vi "PDash Add Helper Loop.vi"(8 "error in":errorcluster, 10 "Current Selection":T1, 11 "Project":refnum<class "Project.lvclass">) -> (0 "error out":errorcluster, 2 "Current Selection Out":T1, 3 "Project Out":refnum<class "Project.lvclass">)   [LabVIEW 2020, in "Panther Dashboard.lvlib"]
doc: "Panther Dashboard DQMH UI Template"
uses:
  Panther Dashboard.lvlib
  Class/Project/Project.lvclass
  Class/Library/Library.lvclass
  Class/VI/VI.lvclass
  <vilib>/Delacor/Delacor QMH/Libraries/_Scripting Support/Module Type--enum.ctl
  <vilib>/Delacor/Delacor QMH/Libraries/_Scripting Support/dqmh_lib_DQMH Scripting Support.lvlib
  <vilib>/Delacor/Delacor QMH/Libraries/_Scripting Support/Module Info--cluster.ctl
  Controls/Cancel.ctl
  Controls/Continue.ctl
  Controls/Listbox.ctl
panel:
  in  "Current Helper Loops":T2
  out "Selected Module":string caption="Current Module Selection:"
  in  "Helper Loop Name":string
  in  "Continue":T3
  in  "Cancel":T4
  # "Note: To Select the DQMH Default UIs, click the Gear Icon on the Panther Dashboard\nMain UI, and Uncheck the 'Use Panther Dashboard UIs' checkbox."
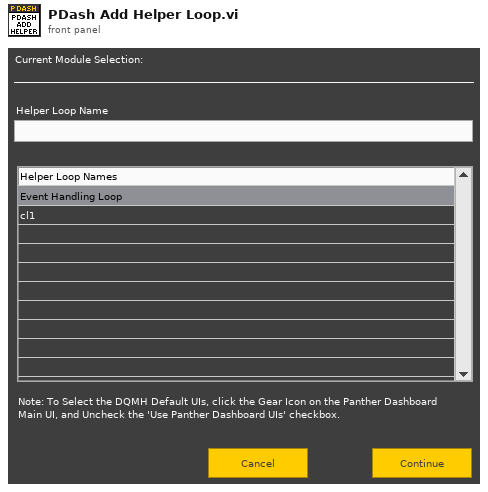
[diagram p1: front panel]
types:
  T1 = cluster{"Library":refnum<class "Library.lvclass">, "VI":refnum<class "VI.lvclass">}
  T2 = typedef "Listbox.ctl" = i32
  T3 = typedef "Continue.ctl" = bool
  T4 = typedef "Cancel.ctl" = bool
  T5 = typedef "dqmh_lib_DQMH Scripting Support.lvlib/Module Info--cluster.ctl" = cluster{"Name":string, "Library":refnum<vi>, "Library Owning App":refnum<vi>, "Library Owning Folder":path, "Module Type":T6, "Public API Requests Folder":refnum<vi>, "Public API Requests Arguments Folder":refnum<vi>, "Broadcasts Folder":refnum<vi>, "Broadcasts Arguments Folder":refnum<vi>, "Obtain Broadcast Events VI":refnum<vi>, "Destroy Broadcast Events VI":refnum<vi>, "Obtain Request Events VI":refnum<vi>, "Destroy Request Events VI":refnum<vi>, "Request Events Cluster CTL":refnum<vi>, "Broadcast Events Cluster CTL":refnum<vi>, "Module Timeout VI":refnum<vi>, "Module Name VI":refnum<vi>, "Status Updated VI":refnum<vi>, "Module Not Running Error Constant VI":refnum<vi>}
  T6 = typedef "dqmh_lib_DQMH Scripting Support.lvlib/Module Type--enum.ctl" = enum16{"Singleton", "Cloneable"}
  T7 = typedef "Panther Dashboard.lvlib/Module type--enum.ctl" = enum16{"Singleton", "Cloneable"}
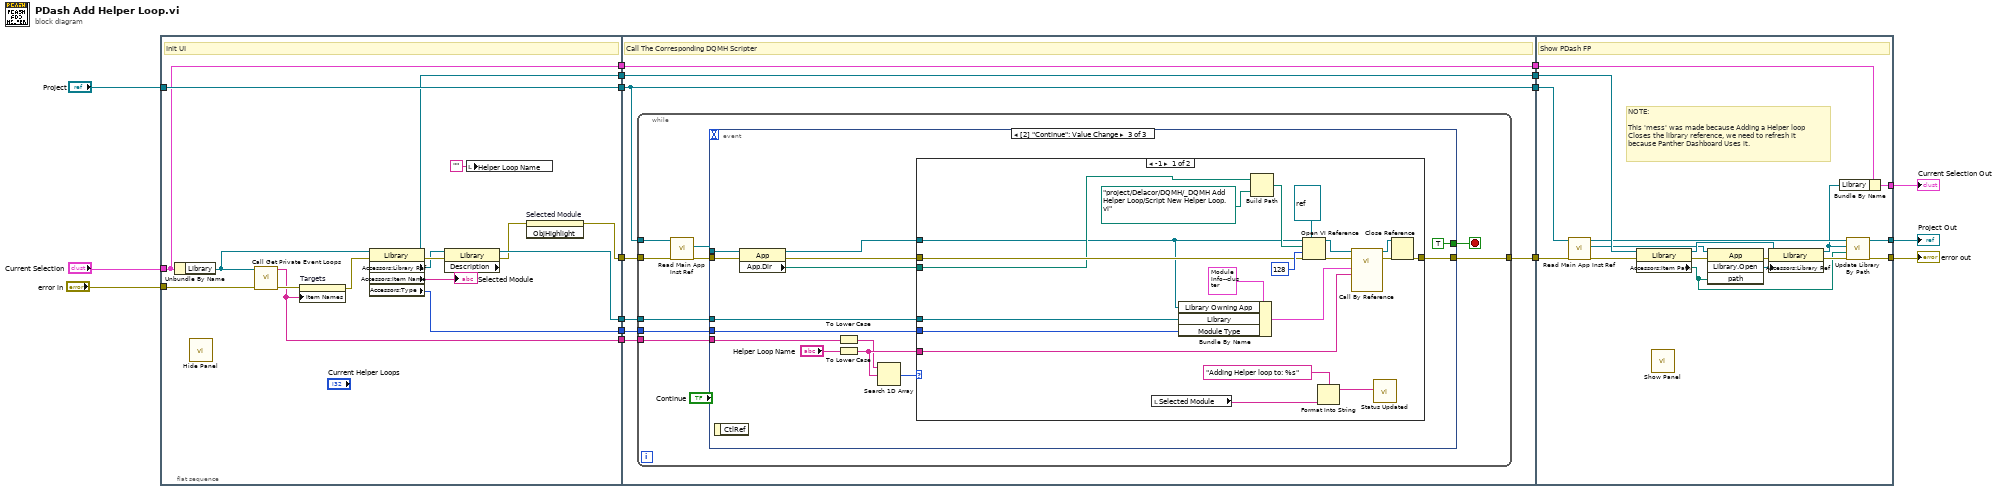
[diagram p0: block diagram]
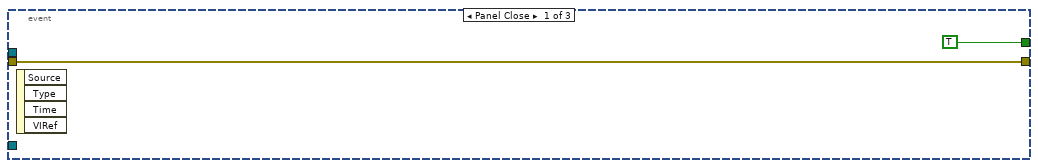
[diagram p2: hidden frame]
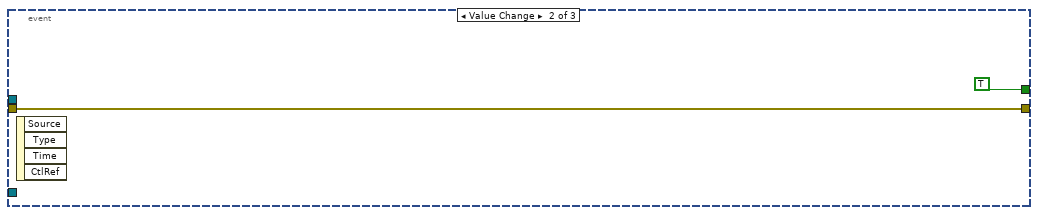
[diagram p3: hidden frame]
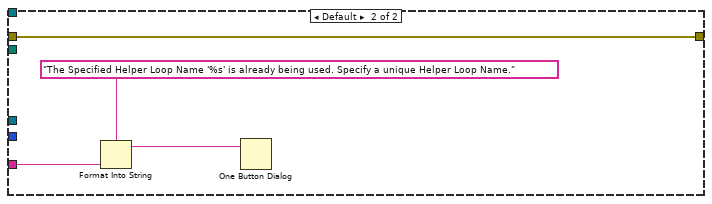
[diagram p4: hidden frame]
diagram:
  n1 = flat-sequence {
    tunnel: "Project" -> [w32]
    tunnel: [w32] -> w13
    tunnel: "error in" -> [w25]
    tunnel: [w26] -> w15
    tunnel: "Current Selection" -> [w20]
    tunnel: [w29] -> w11
    tunnel: [w22] -> w10
    tunnel: [w21] -> w9
    tunnel: [w20] -> w6
    tunnel: [w18] -> w4
    tunnel: [w41] -> w17
    tunnel: w13 -> [w34]
    tunnel: w15 -> [w40]
    tunnel: w11 -> [w39]
    tunnel: w10 -> [w38]
    tunnel: w9 -> [w37]
    tunnel: [w36] -> w7
    tunnel: w6 -> [w36]
    tunnel: w4 -> [w35]
    tunnel: [w35] -> w3
    tunnel: [w34] -> w1
    tunnel: [w100] -> w8
    tunnel: w17 -> [w97]
    tunnel: [w108] -> w5
    tunnel: w7 -> [w109]
    tunnel: w3 -> [w104]
    tunnel: [w102] -> w2
    tunnel: w1 -> [w93]
    frame #0 {
      # "Init UI"
      n2 = Unbundle By Name(w20) -> ("Library"=w19:refnum<class "Library.lvclass">)
      n3 = call "Hide Panel.vi"() -> ()  [unwired: 11 in, 1 out]
      n4 = call "Call Get Private Event Loops.vi"("error in"=w25, "Library"=w19) -> ("error out"=w24:errorcluster, "Consuming Loop Names"=w22:string[])  [unwired: 7 in, 1 out]
      n5 = property on="Targets" class="LstBox (strict)"(error in=w24, "Item Names"=w22) -> (error out=w23:errorcluster)  [unwired: 1 in, 1 out]
      n6 = property class="Library"(reference=w19, error in=w23) -> (reference out=w18:refnum<class "Library.lvclass">, error out=w33:errorcluster, "Accessors:Library Ref"=w30:refnum<vi>, "Accessors:Item Name"=→"Selected Module":string, "Accessors:Type"=w21:T7)
      n7 = property class="Library" props=["Description"](reference=w30, error in=w33) -> (reference out=w29:refnum<vi>, error out=w27:errorcluster)  [unwired: 1 out]
      n8 = local write "Helper Loop Name"("") -> ()
      n9 = invoke on="Selected Module" class="Str" method="ObjHighlight"(error in=w27) -> (error out=w26:errorcluster)  [unwired: 2 in, 2 out]
    }
    frame #1 {
      # "Call The Corresponding DQMH Scripter"
      n10 = while {
        tunnel: [w48] -> w41
        tunnel: w34 -> [w45]
        tunnel: w40 -> [w43]
        tunnel: w39 -> [w49]
        tunnel: w38 -> [w47]
        tunnel: w37 -> [w46]
        stop <- w50 stop-if-true
        n11 = call "Read Main App Inst Ref.vi"("error in (no error)"=w43, "Project in"=w45) -> ("error out"=w42:errorcluster, "Main App Inst Ref"=w44:refnum<vi>)  [unwired: 7 in, 1 out]
        n12 = event shown="[2] \"Continue\": Value Change" {
          selector: _ -> [_ _ _]
          dyn-events: _ -> [_ _ _]
          timeout: _ -> [_ _ _]
          tunnel: [TRUE TRUE TRUE] -> w50
          tunnel: [w51 w53 w60] -> w48
          tunnel: w42 -> [w51 w53 w59]
          tunnel: w49 -> [_ _ w67]
          tunnel: w47 -> [_ _ w66]
          tunnel: w46 -> [_ _ w63]
          tunnel: w44 -> [_ _ w55]
          event Panel Close {
            n13 = event-data() -> ()  [unwired: 1 in, 4 out]
          }
          event Value Change {
            n14 = event-data() -> ()  [unwired: 1 in, 4 out]
          }
          event Value Change {
            n15 = event-data() -> ()  [unwired: 1 in, 1 out]
            n16 = property class="App"(reference=w55, error in=w59) -> (reference out=w58:refnum<vi>, error out=w57:errorcluster, "App.Dir"=w56:path)
            n17 = To Lower Case(string=w66) -> (all lower case string=w64:string[])
            n18 = To Lower Case(string="Helper Loop Name") -> (all lower case string=w65:string)
            n19 = Search 1D Array(1D array=w64, element=w65) -> (index of element=w61:i32)  [unwired: 1 in]
            n20 = case shown="-1" w61 {
              tunnel: w67 -> [w81 _]
              tunnel: [w77 w89] -> w60
              tunnel: w65 -> [w76 w92]
              tunnel: w63 -> [w75 _]
              tunnel: w58 -> [w69 _]
              tunnel: w57 -> [w71 w89]
              tunnel: w56 -> [w70 _]
              frame -1 {
                n21 = local read "Selected Module"() -> (w72:string)
                n22 = Bundle By Name(cluster=T5 {"Name"="", "Library"=refnum, "Library Owning App"=refnum, "Library Owning Folder"=path "", "Module Type"=enum."Singleton", "Public API Requests Folder"=refnum, "Public API Requests Arguments Folder"=refnum, "Broadcasts Folder"=refnum, "Broadcasts Arguments Folder"=refnum, "Obtain Broadcast Events VI"=refnum, "Destroy Broadcast Events VI"=refnum, "Obtain Request Events VI"=refnum, "Destroy Request Events VI"=refnum, "Request Events Cluster CTL"=refnum, "Broadcast Events Cluster CTL"=refnum, "Module Timeout VI"=refnum, "Module Name VI"=refnum, "Status Updated VI"=refnum, "Module Not Running Error Constant VI"=refnum} ("Module Info in"), "Library Owning App"=w69, "Library"=w81, "Module Type"=w75) -> (w86:T5)
                n23 = Build Path(base path=w70, name or relative path=path "project/Delacor/DQMH/_DQMH Add Helper Loop/Script New Helper Loop.vi") -> (appended path=w85:path)
                n24 = Open VI Reference(type specifier VI Refnum (for type only)=refnum<vi> refnum, application reference (local)=w69, vi path=w85, options=128, error in (no error)=w71) -> (vi reference=w88:refnum<vi>, error out=w83:errorcluster)  [unwired: 1 in]
                n25 = Format Into String(format string="Adding Helper loop to: %s" ("Status"), w72) -> (resulting string=w74:string)  [unwired: 2 in, 1 out]
                n26 = call-by-ref "?"(reference=w88, error in=w83, "New Helper Loop Name"=w76, "Module Info"=w86) -> (reference out=w87:refnum<vi>, error out=w84:errorcluster)  [unwired: 9 in, 1 out]
                n27 = call "Status Updated.vi"("Status"=w74) -> ()  [unwired: 10 in, 1 out]
                n28 = Close Reference(reference=w87, error in (no error)=w84) -> (error out=w77:errorcluster)
              }
              frame Default {
                n29 = Format Into String(format string="The Specified Helper Loop Name '%s' is already being used. Specify a unique Helper Loop Name.", w92) -> (resulting string=w91:string)  [unwired: 2 in, 1 out]
                n30 = One Button Dialog(message=w91) -> ()  [unwired: 1 in, 1 out]
              }
            }
          }
        }
      }
    }
    frame #2 {
      # "NOTE:\n\nThis 'mess' was made because Adding a Helper loop\nCloses the library reference, we need to refresh it\nbecause Panther Dashboard Uses it."
      # "Show PDash FP"
      n31 = call "Read Main App Inst Ref.vi"("error in (no error)"=w97, "Project in"=w93) -> ("error out"=w96:errorcluster, "Main App Inst Ref"=w98:refnum<vi>, "Project out"=w99:refnum<class "Project.lvclass">)  [unwired: 7 in]
      n32 = property class="Library"(reference=w104, error in=w96) -> (reference out=w103:refnum<class "Library.lvclass">, error out=w105:errorcluster, "Accessors:Item Path"=w94:path)
      n33 = call "Show Panel.vi"() -> ()  [unwired: 11 in, 1 out]
      n34 = invoke class="App" method="Library.Open"(reference=w98, error in=w105, "path"=w94) -> (error out=w107:errorcluster, "Open Library"=w106:refnum<vi>)  [unwired: 1 in, 2 out]
      n35 = property class="Library"(reference=w103, error in=w107, "Accessors:Library Ref"=w106) -> (reference out=w95:refnum<class "Library.lvclass">, error out=w101:errorcluster)
      n36 = Bundle By Name(cluster=w109, "Library"=w95) -> (w108:T1)
      n37 = call "Update Library By Path.vi"("error in"=w101, "Library Path to be Replaced"=w94, "Library"=w95, "Project in"=w99) -> ("error out"=w100:errorcluster, "Project out"=w102:refnum<class "Project.lvclass">)  [unwired: 6 in]
    }
  }
  "error out" <- w8
  "Current Selection Out" <- w5
  "Project Out" <- w2
